vi "Register Dynamic Events.vi"(8 "error in (no error)":errorcluster, 11 "TreeControlEventHandler In":refnum<class "TreeControlEventHandler.lvclass">) -> (0 "error out":errorcluster, 3 "TreeControlEventHandler Out":refnum<class "TreeControlEventHandler.lvclass">)   [LabVIEW 2015, in "ActorEvents.lvlib" / "TreeControlEventHandler.lvclass"]
uses:
  TreeControlEventHandler.lvclass
  IEventHandler/IEventHandler.lvclass
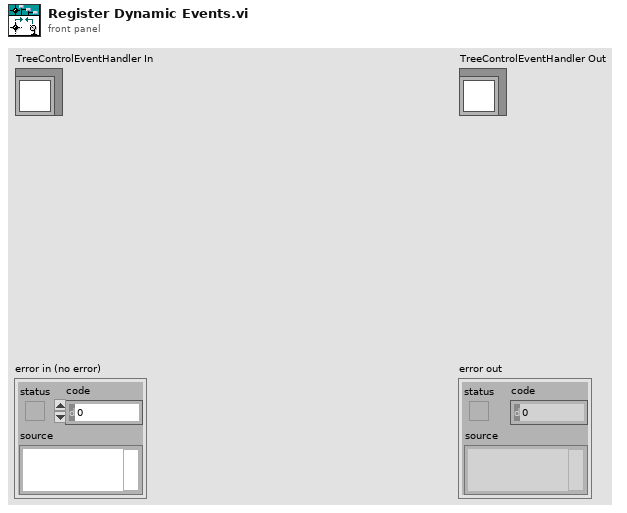
[diagram p1: front panel]
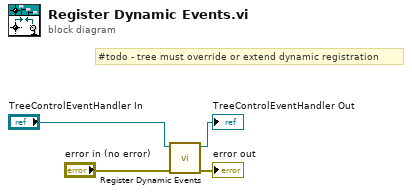
[diagram p0: block diagram]
diagram:
  # "#todo - tree must override or extend dynamic registration"
  n1 = call-parent "Register Dynamic Events.vi"("error in (no error)"="error in (no error)", "IEventHandler In"="TreeControlEventHandler In") -> ("error out"=→"error out":errorcluster, "IEventHandler Out"=→"TreeControlEventHandler Out":refnum<class "TreeControlEventHandler.lvclass">)  [unwired: 8 in]
